vi "Q_Driver.vi"(0 "Q_Name":string, 1 "State":string, 2 "States[]":string[](array[string]), 11 "error in (no error)":errorcluster, 13 "Q_Operation":T1) -> (3 "Queue Elements":string[](array[string]), 4 "State Out":string, 15 "error out":errorcluster)   [LabVIEW 2020]
uses:
  Typedefs/Q_operation.ctl
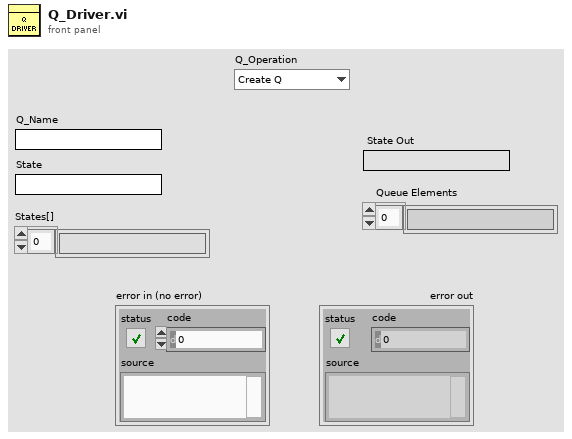
[diagram p1: front panel]
types:
  T1 = typedef "Q_operation.ctl" = enum16{"Create Q", "Enqueue 1", "Enqueue N", "Enstack 1", "Enstack N", "Dequeue", "Flush", "Release", "Preview"}
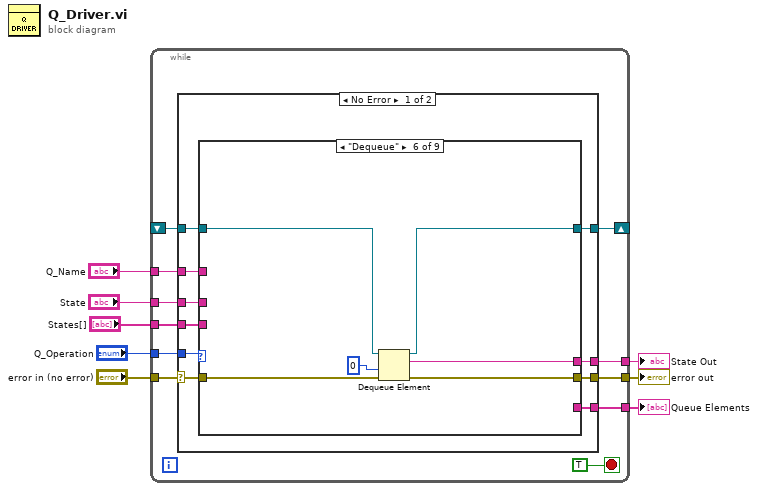
[diagram p0: block diagram]
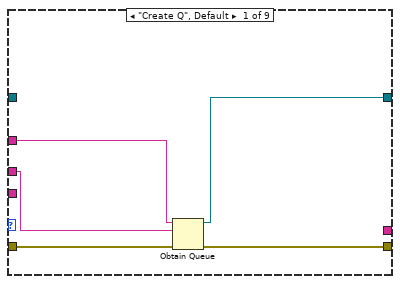
[diagram p2: hidden frame]
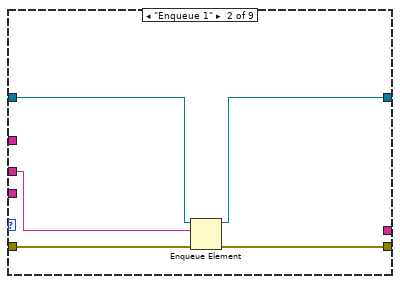
[diagram p3: hidden frame]
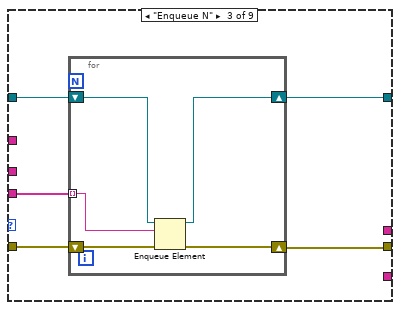
[diagram p4: hidden frame]
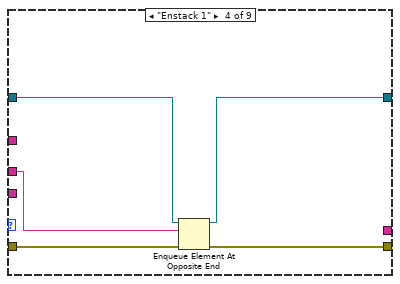
[diagram p5: hidden frame]
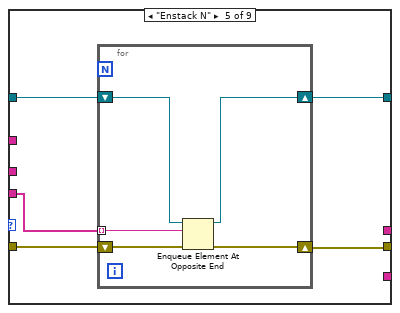
[diagram p6: hidden frame]
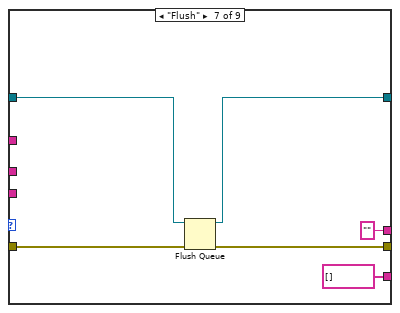
[diagram p7: hidden frame]
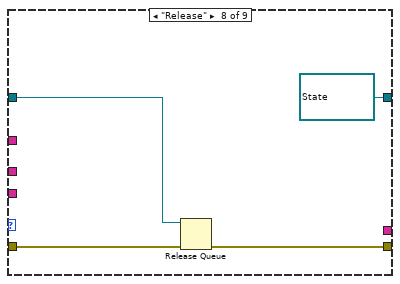
[diagram p8: hidden frame]
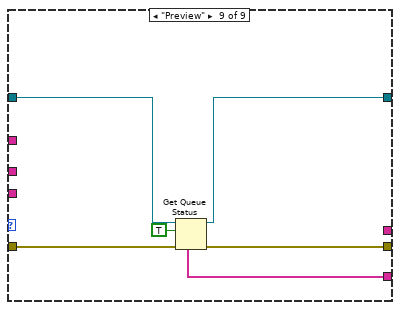
[diagram p9: hidden frame]
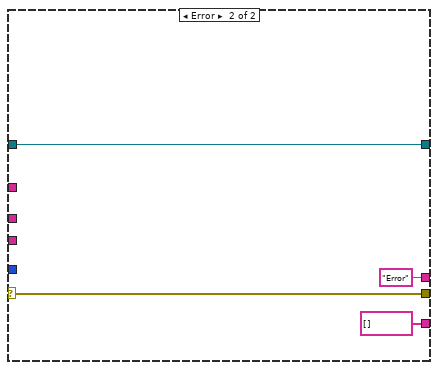
[diagram p10: hidden frame]
diagram:
  n1 = while {
    tunnel: "error in (no error)" -> [w19]
    tunnel: [w18] -> w7
    tunnel: "Q_Operation" -> [w17]
    tunnel: "Q_Name" -> [w16]
    tunnel: "State" -> [w15]
    shift-right: [w14] -> _
    shift-left: _ -> [w13]
    tunnel: [w12] -> w3
    tunnel: [w11] -> w2
    tunnel: "States[]" -> [w10]
    stop <- TRUE stop-if-true
    n2 = case shown="No Error" w19 {
      selector: w19 -> [w29 w88]
      tunnel: [w28 w88] -> w18
      tunnel: w17 -> [w27 _]
      tunnel: w16 -> [w26 _]
      tunnel: w15 -> [w25 _]
      tunnel: [w24 w90] -> w14
      tunnel: w13 -> [w23 w90]
      tunnel: [w22 string[] [] ("elements")] -> w12
      tunnel: [w21 "Error" ("State")] -> w11
      tunnel: w10 -> [w20 _]
      frame No Error {
        n3 = case shown="\"Dequeue\"" w27 {
          tunnel: [w34 w39 w43 w54 w58 w70 w76 w80 w86] -> w28
          tunnel: w29 -> [w33 w38 w44 w53 w59 w69 w75 w79 w85]
          tunnel: w26 -> [w32 _ _ _ _ _ _ _ _]
          tunnel: w25 -> [w31 w35 _ w52 _ _ _ _ _]
          tunnel: [w30 w36 w42 w50 w56 w68 w73 refnum<queue> refnum ("queue out") w83] -> w24
          tunnel: w23 -> [_ w37 w41 w51 w57 w67 w74 w78 w84]
          tunnel: [_ _ _ _ _ _ string[] [] ("elements") _ w81] -> w22
          tunnel: [_ _ _ _ _ w65 "" ("State") _ _] -> w21
          tunnel: w20 -> [_ _ w40 _ w55 _ _ _ _]
          frame "Create Q", Default {
            n4 = Obtain Queue(name (unnamed)=w32, element data type=w31, error in (no error)=w33) -> (queue out=w30:refnum<queue>, error out=w34:errorcluster)  [unwired: 2 in, 1 out]
          }
          frame "Enqueue 1" {
            n5 = Enqueue Element(queue=w37, element=w35, error in (no error)=w38) -> (queue out=w36:refnum<queue>, error out=w39:errorcluster)  [unwired: 1 in, 1 out]
          }
          frame "Enqueue N" {
            n6 = for {
              shift-right: [w48] -> w43
              shift-left: w44 -> [w49]
              shift-right: [w47] -> w42
              shift-left: w41 -> [w46]
              tunnel: w40 -> [w45] mode=indexing
              n7 = Enqueue Element(queue=w46, element=w45, error in (no error)=w49) -> (queue out=w47:refnum<queue>, error out=w48:errorcluster)  [unwired: 1 in, 1 out]
            }
          }
          frame "Enstack 1" {
            n8 = Enqueue Element At Opposite End(queue=w51, element=w52, error in (no error)=w53) -> (queue out=w50:refnum<queue>, error out=w54:errorcluster)  [unwired: 1 in, 1 out]
          }
          frame "Enstack N" {
            n9 = for {
              shift-right: [w63] -> w58
              shift-left: w59 -> [w64]
              shift-right: [w61] -> w56
              shift-left: w57 -> [w62]
              tunnel: w55 -> [w60] mode=indexing
              n10 = Enqueue Element At Opposite End(queue=w62, element=w60, error in (no error)=w64) -> (queue out=w61:refnum<queue>, error out=w63:errorcluster)  [unwired: 1 in, 1 out]
            }
          }
          frame "Dequeue" {
            n11 = Dequeue Element(queue=w67, timeout in ms (-1)=0, error in (no error)=w69) -> (queue out=w68:refnum<queue>, element=w65:string, error out=w70:errorcluster)  [unwired: 1 out]
          }
          frame "Flush" {
            n12 = Flush Queue(queue=w74, error in (no error)=w75) -> (queue out=w73:refnum<queue>, error out=w76:errorcluster)  [unwired: 1 out]
          }
          frame "Release" {
            n13 = Release Queue(queue=w78, error in (no error)=w79) -> (error out=w80:errorcluster)  [unwired: 1 in, 2 out]
          }
          frame "Preview" {
            n14 = Get Queue Status(queue=w84, return elements? (F)=TRUE, error in (no error)=w85) -> (queue out=w83:refnum<queue>, error out=w86:errorcluster, elements=w81:string[])  [unwired: 5 out]
          }
        }
      }
      frame Error {
      }
    }
  }
  "error out" <- w7
  "Queue Elements" <- w3
  "State Out" <- w2
